vi "[FP] - Set Front Panel to position if enabled.vi"(6 "App Kind":T4(ring), 7 "Show":bool, 8 "Error":errorcluster, 9 "Vi To Move Settings":T2={"Menu Bar"=FALSE, "Position"=enum."MID-CTR", "border(px)"=-2, "Monitor #"=0}, 10 "Postion":T1, 11 "VI To Move":refnum<vi>) -> (0 "Error Out":errorcluster)   [LabVIEW 2015]
uses:
  TypeDefs_Utility/Cluster_FP_Position  and Size Data.ctl
  TypeDefs_Utility/ENUM RB_Pos_Quadrant Position.ctl
  TypeDefs_Utility/Cluster_Pos_Top Left position.ctl
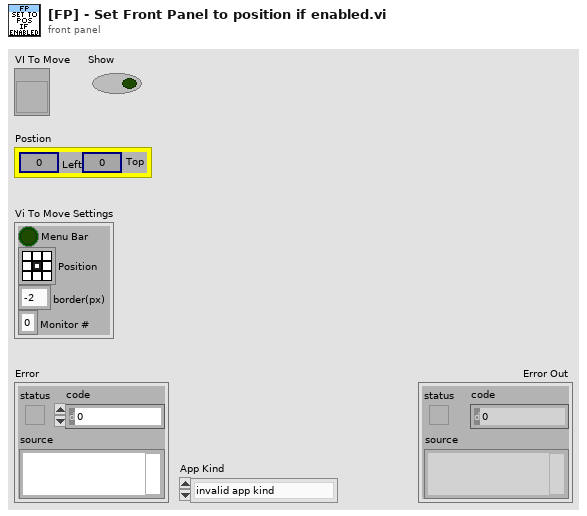
[diagram p1: front panel]
types:
  T1 = typedef "Cluster_Pos_Top Left position.ctl" = cluster{"Left":i16, "Top":i16}
  T2 = typedef "Cluster_FP_Position  and Size Data.ctl" = cluster{"Menu Bar":bool, "Position":T3, "border(px)":i32, "Monitor #":u16}
  T3 = typedef "ENUM RB_Pos_Quadrant Position.ctl" = enum32{"LFT-TOP", "MID-TOP", "RGT-TOP", "LFT-CTR", "MID-CTR", "RGT-CTR", "LFT-BOT", "MID-BOT", "RGT-BOT"}
  T4 = enum32{"invalid app kind", "Development System", "Run Time System", "Student Edition", "Embedded LabVIEW", "Evaluation", "Custom"}
  T5 = enum32{"Invalid", "Standard", "Closed", "Hidden", "Minimized", "Maximized"}
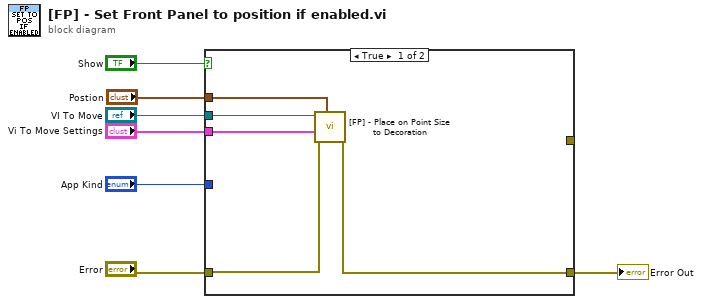
[diagram p0: block diagram]
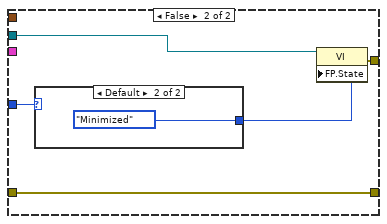
[diagram p2: hidden frame]
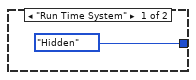
[diagram p3: hidden frame]
diagram:
  n1 = case shown="True" "Show" {
    tunnel: "Error" -> [w12 w13]
    tunnel: [w11 w13] -> w5
    tunnel: "VI To Move" -> [w10 w16]
    tunnel: "App Kind" -> [_ w17]
    tunnel: [_ w14] -> _
    tunnel: "Vi To Move Settings" -> [w9 _]
    tunnel: "Postion" -> [w8 _]
    frame True {
      n2 = call "[FP] - Place on Point Size to Decoration.vi"("Point"=w8, "Error"=w12, "FPSet"=w9, "VI Ref"=w10) -> ("Error Out"=w11:errorcluster)  [unwired: 6 in, 1 out]
    }
    frame False {
      n3 = case shown="Default" w17 {
        tunnel: [T5."Hidden" ("Front Panel Window:State") T5."Minimized" ("Front Panel Window:State")] -> w15
        frame "Run Time System" {
        }
        frame Default {
        }
      }
      n4 = property class="VI"(reference=w16, "FP.State"=w15) -> (error out=w14:errorcluster)  [unwired: 1 in, 1 out]
    }
  }
  "Error Out" <- w5
